vi "Uses Buffer.vi"(8 "error in (no error)":errorcluster, 11 "Driver in":refnum<class "Driver.lvclass">) -> (0 "error out":errorcluster, 2 "Uses Buffer":bool, 3 "Driver out":refnum<class "Driver.lvclass">)   [LabVIEW 2023, in "HAF.lvlib" / "Driver.lvclass"]
doc: "Indicates whether or not this Driver interfaces with an instrument that uses a Buffer to store results (it may be called something different.) This will be used as part of command construction.\n\nThe default is to return False; subclasses should override as necessary."
uses:
  Driver.lvclass
  Driver.lvclass/Driver.ctl
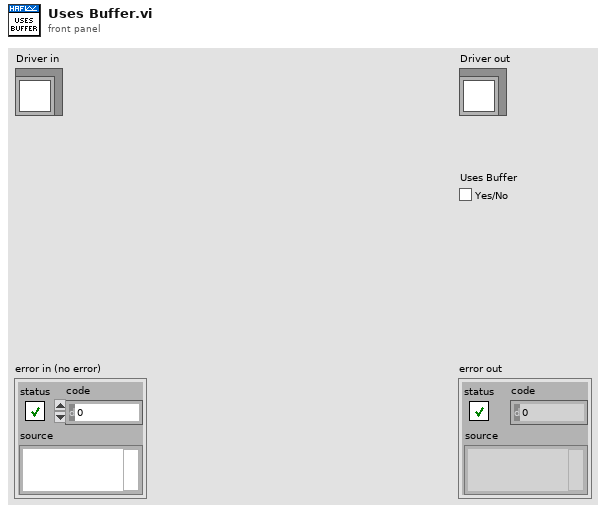
[diagram p1: front panel]
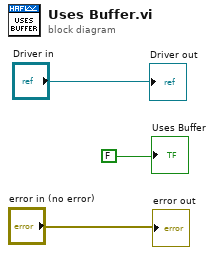
[diagram p0: block diagram]
diagram:
  "error out" <- "error in (no error)"
  "Driver out" <- "Driver in"
  "Uses Buffer" <- FALSE
